vi "SetResult.vi"(0 "TestMeasureStep in":refnum<class "TestMeasureStep.lvclass">, 5 "StringMeas":string, 7 "Meas":dbl, 11 "error in (no error)":errorcluster, 12 "Use Error As result":bool) -> (4 "TestMeasureStep out":refnum<class "TestMeasureStep.lvclass">, 8 "TestStatus":T1, 15 "error out":errorcluster)   [LabVIEW 2019, in "TestMeasureStep.lvclass"]
uses:
  TestMeasureStep.lvclass
  testSeq/Typedef/TestStatus.ctl
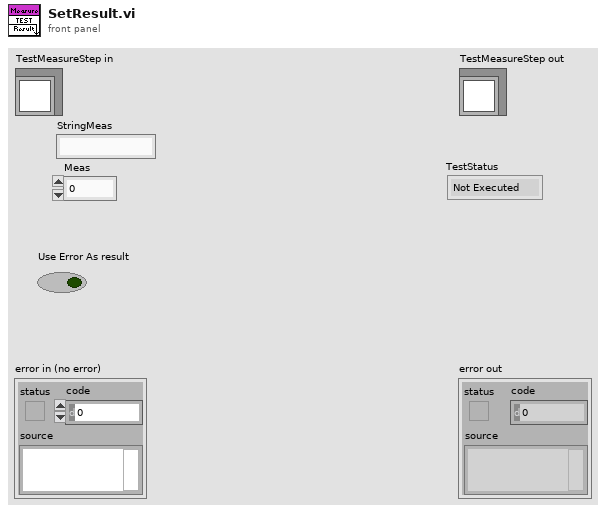
[diagram p1: front panel]
types:
  T1 = typedef "TestStatus.ctl" = enum16{"Not Executed", "Passed", "Failed", "Inconclusive", "Processing"}
  T2 = typedef "TestSeqClass.lvclass/TesstepType.ctl" = cluster{"TestName":string, "Meas":dbl, "Min ":dbl, "Max":dbl, "TestStatus":T1, "StringLimit":string, "StringMeas":string, "Unit":string}
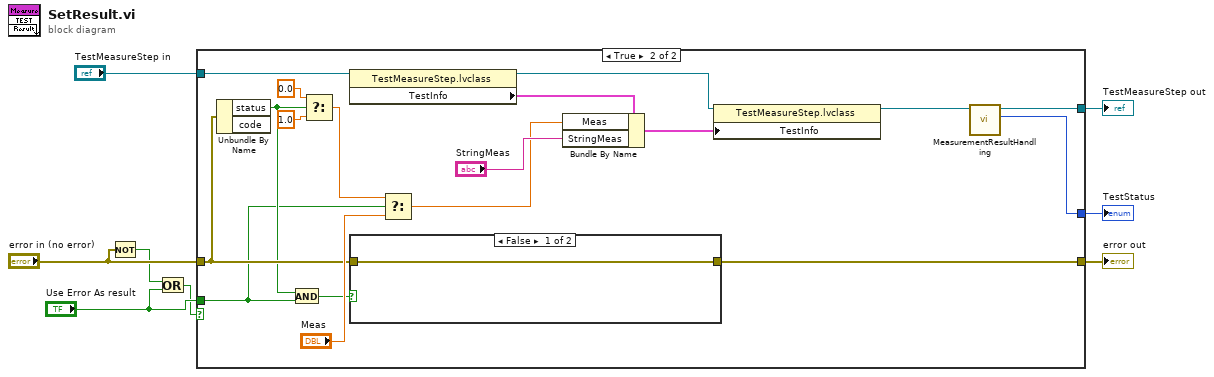
[diagram p0: block diagram]
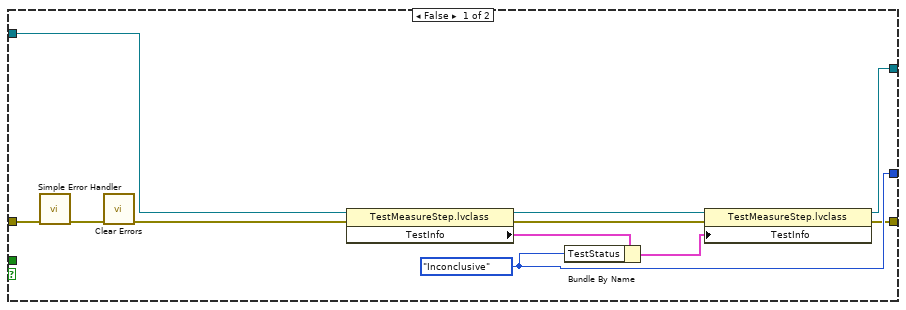
[diagram p2: hidden frame]
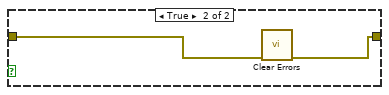
[diagram p3: hidden frame]
diagram:
  n1 = Not(x="error in (no error)") -> (.not. x?=w2:bool)
  n2 = Or(x=w2, y="Use Error As result") -> (x .or. y?=w4:bool)
  n3 = case shown="True" w4 {
    tunnel: [w14 w37] -> w8
    tunnel: [w18 w35] -> w7
    tunnel: "Use Error As result" -> [_ w20]
    tunnel: "error in (no error)" -> [w13 w28]
    tunnel: [w9 w27] -> w6
    tunnel: "TestMeasureStep in" -> [w17 w25]
    frame False {
      w18 = TestStatus."Inconclusive" ("TestStatus")
      n4 = call <vilib>:"Simple Error Handler.vi"("error in (no error)"=w13) -> ("error out"=w12:errorcluster)  [unwired: 4 in, 4 out]
      n5 = call <vilib>:"Clear Errors.vi"("error in (no error)"=w12) -> ("error out"=w11:errorcluster)  [unwired: 5 in, 1 out]
      n6 = property class="TestMeasureStep.lvclass"(reference=w17, error in=w11) -> (reference out=w15:refnum<class "TestMeasureStep.lvclass">, error out=w10:errorcluster, "TestInfo"=w19:T2)
      n7 = Bundle By Name(cluster=w19, "TestStatus"=w18) -> (w16:T2)
      n8 = property class="TestMeasureStep.lvclass"(reference=w15, error in=w10, "TestInfo"=w16) -> (reference out=w14:refnum<class "TestMeasureStep.lvclass">, error out=w9:errorcluster)
    }
    frame True {
      n9 = Unbundle By Name(w28) -> ("status"=w24:bool)  [unwired: 1 out]
      n10 = And(x=w24, y=w20) -> (x .and. y?=w26:bool)
      n11 = Select(t=0.0, s=w24, f=1.0) -> (s? t:f=w21:dbl)
      n12 = property class="TestMeasureStep.lvclass"(reference=w25) -> (reference out=w30:refnum<class "TestMeasureStep.lvclass">, "TestInfo"=w32:T2)  [unwired: 1 in, 1 out]
      n13 = case shown="False" w26 {
        tunnel: w28 -> [w38 w40]
        tunnel: [w38 w39] -> w27
        frame False {
        }
        frame True {
          n14 = call <vilib>:"Clear Errors.vi"("error in (no error)"=w40) -> ("error out"=w39:errorcluster)  [unwired: 5 in, 1 out]
        }
      }
      n15 = Select(t=w21, s=w20, f="Meas") -> (s? t:f=w34:dbl)
      n16 = Bundle By Name(cluster=w32, "Meas"=w34, "StringMeas"="StringMeas") -> (w31:T2)
      n17 = property class="TestMeasureStep.lvclass"(reference=w30, "TestInfo"=w31) -> (reference out=w29:refnum<class "TestMeasureStep.lvclass">)  [unwired: 1 in, 1 out]
      n18 = call "MeasurementResultHandling.vi"("TestMeasureStep in"=w29) -> ("TestStatus"=w35:T1, "TestMeasureStep out"=w37:refnum<class "TestMeasureStep.lvclass">)  [unwired: 8 in, 1 out]
    }
  }
  "error out" <- w6
  "TestMeasureStep out" <- w8
  "TestStatus" <- w7
